vi "VtoT.vi"(1 "Volt":dbl) -> (0 "Temp":dbl)   [LabVIEW 2016]
doc: "Подпрограмма предназначена для перевода считанного с DAQ\nнапряжения в диапазоне 1-5В в температуру в диап. 0-40оС"
panel:
  # "Подпрограмма предназначена для перевода считанного с DAQ\nнапряжения в диапазоне 1-5В в температуру в диап. 0-40оС"
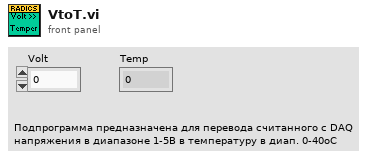
[diagram p1: front panel]
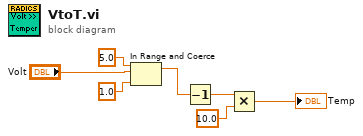
[diagram p0: block diagram]
diagram:
  n1 = In Range and Coerce(upper limit=5.0, x="Volt", lower limit=1.0) -> (coerced(x)=w5:dbl)  [unwired: 1 out]
  n2 = Decrement(x=w5) -> (x-1=w6:dbl)
  n3 = Multiply(x=w6, y=10.0) -> (x*y=→"Temp":dbl)
